vi "CreateTemperatureLogString.vi"(11 "Temperatures (C)":dbl[](array[numeric])) -> (3 "Temperature Log String":string)   [LabVIEW 2012]
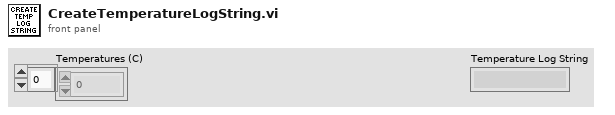
[diagram p1: front panel]
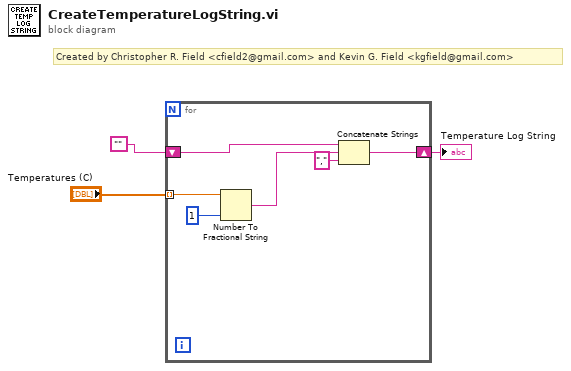
[diagram p0: block diagram]
diagram:
  # "Created by Christopher R. Field <cfield2@gmail.com> and Kevin G. Field <kgfield@gmail.com>"
  n1 = for {
    tunnel: "Temperatures (C)" -> [w9] mode=indexing
    shift-right: [w4] -> w1
    shift-left: "" -> [w7]
    n2 = Number To Fractional String(number=w9, precision (6)=i16 1) -> (F-format string=w6:string)  [unwired: 2 in]
    n3 = Concatenate Strings(w7, w6, "," ("string")) -> (w4:string)
  }
  "Temperature Log String" <- w1
